vi "ShortestPath.vi"() -> ()   [LabVIEW 2009]
uses:
  OccupancyMap/OccupancyMap.lvclass
  OccupancyMap/parameters.ctl
  Rectangle/Rectangle.lvclass
panel:
  in  "Solve":bool
  out "Occupancy Map":picture
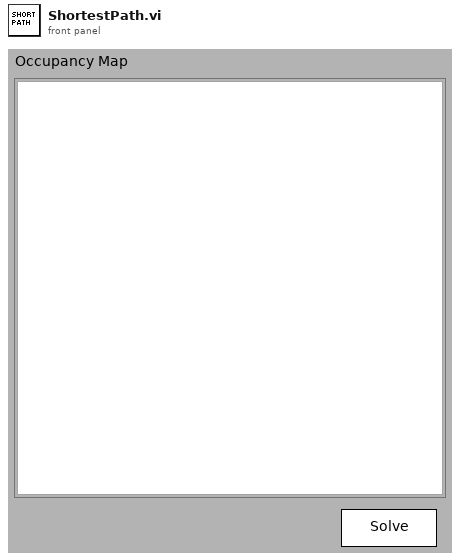
[diagram p1: front panel]
types:
  T1 = cluster{"left":i16, "top":i16, "right":i16, "bottom":i16}
  T2 = cluster{"Left":dbl, "Right":dbl, "Top":dbl, "Bottom":dbl}
  T3 = cluster{"Width":i16, "Style":enum32{"Solid", "Dash", "Dot", "DashDot", "DashDotDot"}}
  T4 = typedef "OccupancyMap.lvclass/parameters.ctl" = cluster{"MapResolution":cluster{"resX":dbl, "resY":dbl}, "StartLocation":cluster{"X":dbl, "Y":dbl}, "Goal":cluster{"X":dbl, "Y":dbl}, "MapBoundaries":cluster{"Left":dbl, "Right":dbl, "Top":dbl, "Bottom":dbl}}
  T5 = cluster{"Width":u16, "Style":enum32{"Solid", "Dash", "Dot", "DashDot", "DashDotDot"}}
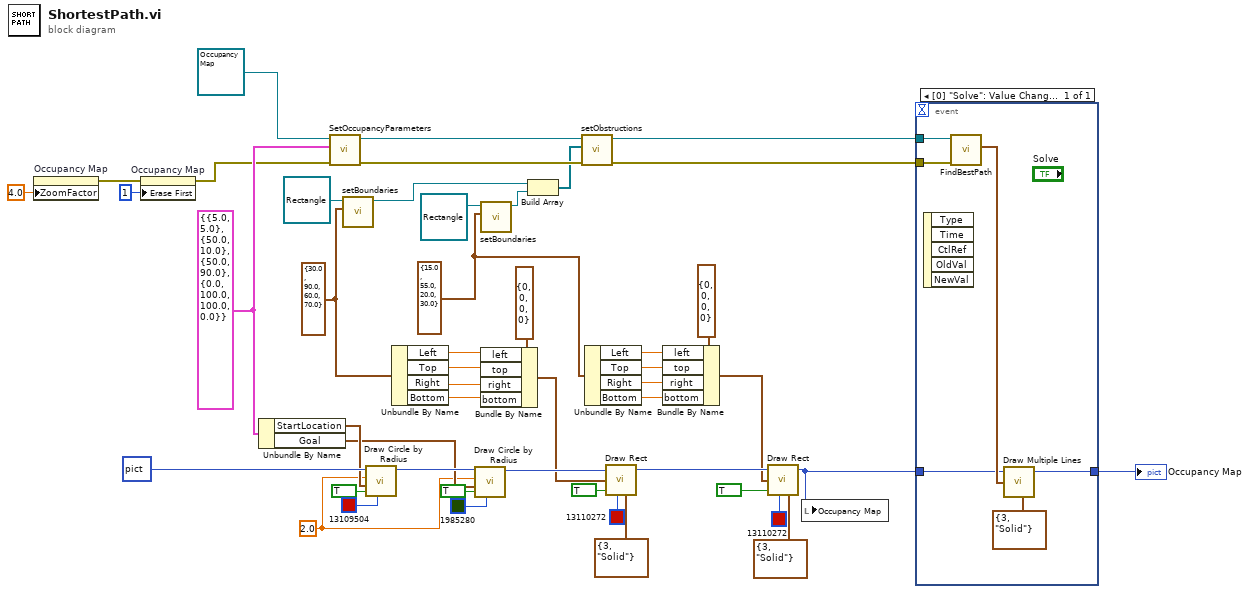
[diagram p0: block diagram]
diagram:
  w7 = T2 {"Left"=15.0, "Right"=55.0, "Top"=20.0, "Bottom"=30.0} ("Boundaries")
  w12 = T2 {"Left"=30.0, "Right"=90.0, "Top"=60.0, "Bottom"=70.0} ("Boundaries")
  w39 = sgl 2.0 ("Zoom Factor")
  w46 = T4 {"MapResolution"={"resX"=5.0, "resY"=5.0}, "StartLocation"={"X"=50.0, "Y"=10.0}, "Goal"={"X"=50.0, "Y"=90.0}, "MapBoundaries"={"Left"=0.0, "Right"=100.0, "Top"=100.0, "Bottom"=0.0}} ("Parameters")
  n1 = property on="Occupancy Map" class="Pict"("ZoomFactor"=sgl 4.0 ("Zoom Factor")) -> (error out=w27:errorcluster)  [unwired: 2 in, 1 out]
  n2 = property on="Occupancy Map" class="Pict"(error in=w27, "Erase First"=u8 1) -> (error out=w26:errorcluster)  [unwired: 1 in, 1 out]
  n3 = Unbundle By Name(w46) -> ("StartLocation"=w45:cluster{"X":dbl, "Y":dbl}, "Goal"=w43:cluster{"X":dbl, "Y":dbl})
  n4 = call "SetOccupancyParameters.vi"("error in (no error)"=w26, "Parameters"=w46, "OccupancyMap in"=refnum<class "OccupancyMap.lvclass"> refnum) -> ("error out"=w35:errorcluster, "OccupancyMap out"=w36:refnum<class "OccupancyMap.lvclass">)  [unwired: 7 in]
  n5 = call "setBoundaries.vi"("Boundaries"=w12, "Rectangle in"=refnum<class "Rectangle.lvclass"> refnum ("Rectangle.lvclass")) -> ("Rectangle out"=w32:refnum<class "Rectangle.lvclass">)  [unwired: 8 in, 1 out]
  n6 = call <vilib>:"Draw Circle by Radius.vi"("color(black)"=u32 13109504, "fill?(F)"=TRUE, "pixel center"=w45, "radius"=w39, "picture"=picture data[5B] ("2D Picture")) -> ("new picture"=w44:picture)  [unwired: 6 in]
  n7 = Unbundle By Name(w12) -> ("Left"=w31:dbl, "Top"=w30:dbl, "Right"=w29:dbl, "Bottom"=w28:dbl)
  n8 = call <vilib>:"Draw Circle by Radius.vi"("color(black)"=u32 1985280, "fill?(F)"=TRUE, "pixel center"=w43, "radius"=w39, "picture"=w44) -> ("new picture"=w22:picture)  [unwired: 6 in]
  n9 = call "setBoundaries.vi"("Boundaries"=w7, "Rectangle in"=refnum<class "Rectangle.lvclass"> refnum ("Rectangle.lvclass")) -> ("Rectangle out"=w10:refnum<class "Rectangle.lvclass">)  [unwired: 8 in, 1 out]
  n10 = Bundle By Name(cluster=T1 {"left"=0, "top"=0, "right"=0, "bottom"=0} ("rect"), "left"=w31, "top"=w30, "right"=w29, "bottom"=w28) -> (w14:T1)
  n11 = Build Array(w32, w10) -> (w34:refnum<class "Rectangle.lvclass">[])
  n12 = call "setObstructions.vi"("error in (no error)"=w35, "Obstructions"=w34, "OccupancyMap in"=w36) -> ("error out"=w38:errorcluster, "OccupancyMap out"=w37:refnum<class "OccupancyMap.lvclass">)  [unwired: 7 in]
  n13 = Unbundle By Name(w7) -> ("Left"=w8:dbl, "Top"=w6:dbl, "Right"=w5:dbl, "Bottom"=w4:dbl)
  n14 = call <vilib>:"Draw Rect.vi"("picture"=w22, "rect"=w14, "fill?(F)"=TRUE, "color(black)"=u32 13110272, "pen"=T3 {"Width"=3, "Style"=enum."Solid"}) -> ("new picture"=w20:picture)  [unwired: 4 in]
  n15 = Bundle By Name(cluster=T1 {"left"=0, "top"=0, "right"=0, "bottom"=0} ("rect"), "left"=w8, "top"=w6, "right"=w5, "bottom"=w4) -> (w3:T1)
  n16 = call <vilib>:"Draw Rect.vi"("picture"=w20, "rect"=w3, "fill?(F)"=TRUE, "color(black)"=u32 13110272, "pen"=T3 {"Width"=3, "Style"=enum."Solid"}) -> ("new picture"=w16:picture)  [unwired: 4 in]
  n17 = local write "Occupancy Map"(w16) -> ()
  n18 = event shown="[0] \"Solve\": Value Change" {
    selector: _ -> [_]
    dyn-events: _ -> [_]
    timeout: _ -> [_]
    tunnel: w38 -> [w53]
    tunnel: w37 -> [w52]
    tunnel: [w50] -> w17
    tunnel: w16 -> [w49]
    event [0] "Solve": Value Change {
      n19 = event-data() -> ()  [unwired: 1 in, 5 out]
      n20 = call "FindBestPath.vi"("error in (no error)"=w53, "OccupancyMap in"=w52) -> ("path"=w54:cluster{"X":dbl, "Y":dbl}[])  [unwired: 6 in, 3 out]
      n21 = call <vilib>:"Draw Multiple Lines.vi"("picture"=w49, "line endpoints"=w54, "pen"=T5 {"Width"=3, "Style"=enum."Solid"}) -> ("new picture"=w50:picture)  [unwired: 6 in]
    }
  }
  "Occupancy Map" <- w17
